vi "regresion_AB.vi"() -> ()   [LabVIEW 2025]
uses:
  <vilib>/Analysis/Matrix/Datatypes/RealMatrix.ctl
  <vilib>/Analysis/baseanly.llb/Mean (DBL).vi
  <vilib>/Analysis/baseanly.llb/Vector x A.vi
  <vilib>/Analysis/baseanly.llb/Real A x B.vi
  <vilib>/Utility/file.llb/Read Delimited Spreadsheet (DBL).vi
  <vilib>/Utility/file.llb/Read Delimited Spreadsheet (string).vi
  <vilib>/Analysis/Matrix/Numeric/Conversions/Array To Matrix - RA.vi
  <vilib>/Analysis/Matrix/Numeric/Add/Add - RM,RM.vi
  <vilib>/Analysis/Matrix/Numeric/Conversions/Matrix To Array - RM.vi
  <vilib>/Analysis/NI_AALBase.lvlib
  <vilib>/Analysis/Matrix/NI_Matrix.lvlib
  <vilib>/ptbypt/NI_PtbyPt.lvlib
panel:
  out "平滑化":dbl[](array[numeric])
  out "output array":dbl[][](array[numeric])
  out "圧力中心列_2":dbl[](graph)
  out "荷重N_2":dbl[](graph)
  out "平均圧力_2":dbl[](graph)
  out "圧力中心列_1":dbl[](graph)
  out "圧力中心行_1":dbl[](graph)
  out "荷重N_1(接触と似た形)":dbl[](graph)
  out "接触%_1":dbl[](graph)
  out "COPY Graph 3":dbl[](graph)
  out "COPX Graph":dbl[](graph)
  out "Real 2D Array":dbl[][](array[numeric])
  out "element 2":dbl
  out "element":dbl
  out "appended array":dbl[](array[numeric])
  out "python成形済み入力":dbl[](array[numeric])
  out "モデルA出力":T1
  out "モデルB入力":T1
  out "モデルB最終出力":T1
  out "Array 4":dbl[][](array[numeric])
  in  "stop":bool
  out "動画終了フラグ":bool
  out "input array":dbl[](array[numeric])
  out "op_magnitude":dbl
  out "steer_COPy":dbl
  out "steer_COPx":dbl
  out "pedal_COPy":dbl
  out "pedal_COPx":dbl
  out "COP_radius":dbl
  out "phys_torsion":dbl
  out "phys_roll":dbl
  out "phys_pitch":dbl
  out "COP_Y_phys":dbl
  out "+LR/2":dbl
  out "-LR/2":dbl
  out "-FR/2":dbl
  out "+FR/2":dbl
  out "COP_X_phys":dbl
  out "W":dbl
  out "ペダル（0index）":dbl[][](array[numeric])
  out "ペダルを踏んだ量 3":dynamicdata(graph)
  out "表示ループ9":i32
  out "緊急停止フラグ":bool
  out "モデルA重み":dbl[][](array[numeric])
  out "モデルAバイアス":dbl[][](array[numeric])
  out "モデルAオーダー":string[][](array[string])
  out "モデルA入力(最初)":dbl[][](array[numeric])
  out "モデルB重み":dbl[][](array[numeric])
  out "モデルBバイアス":dbl[][](array[numeric])
  # "17"
  # "17"
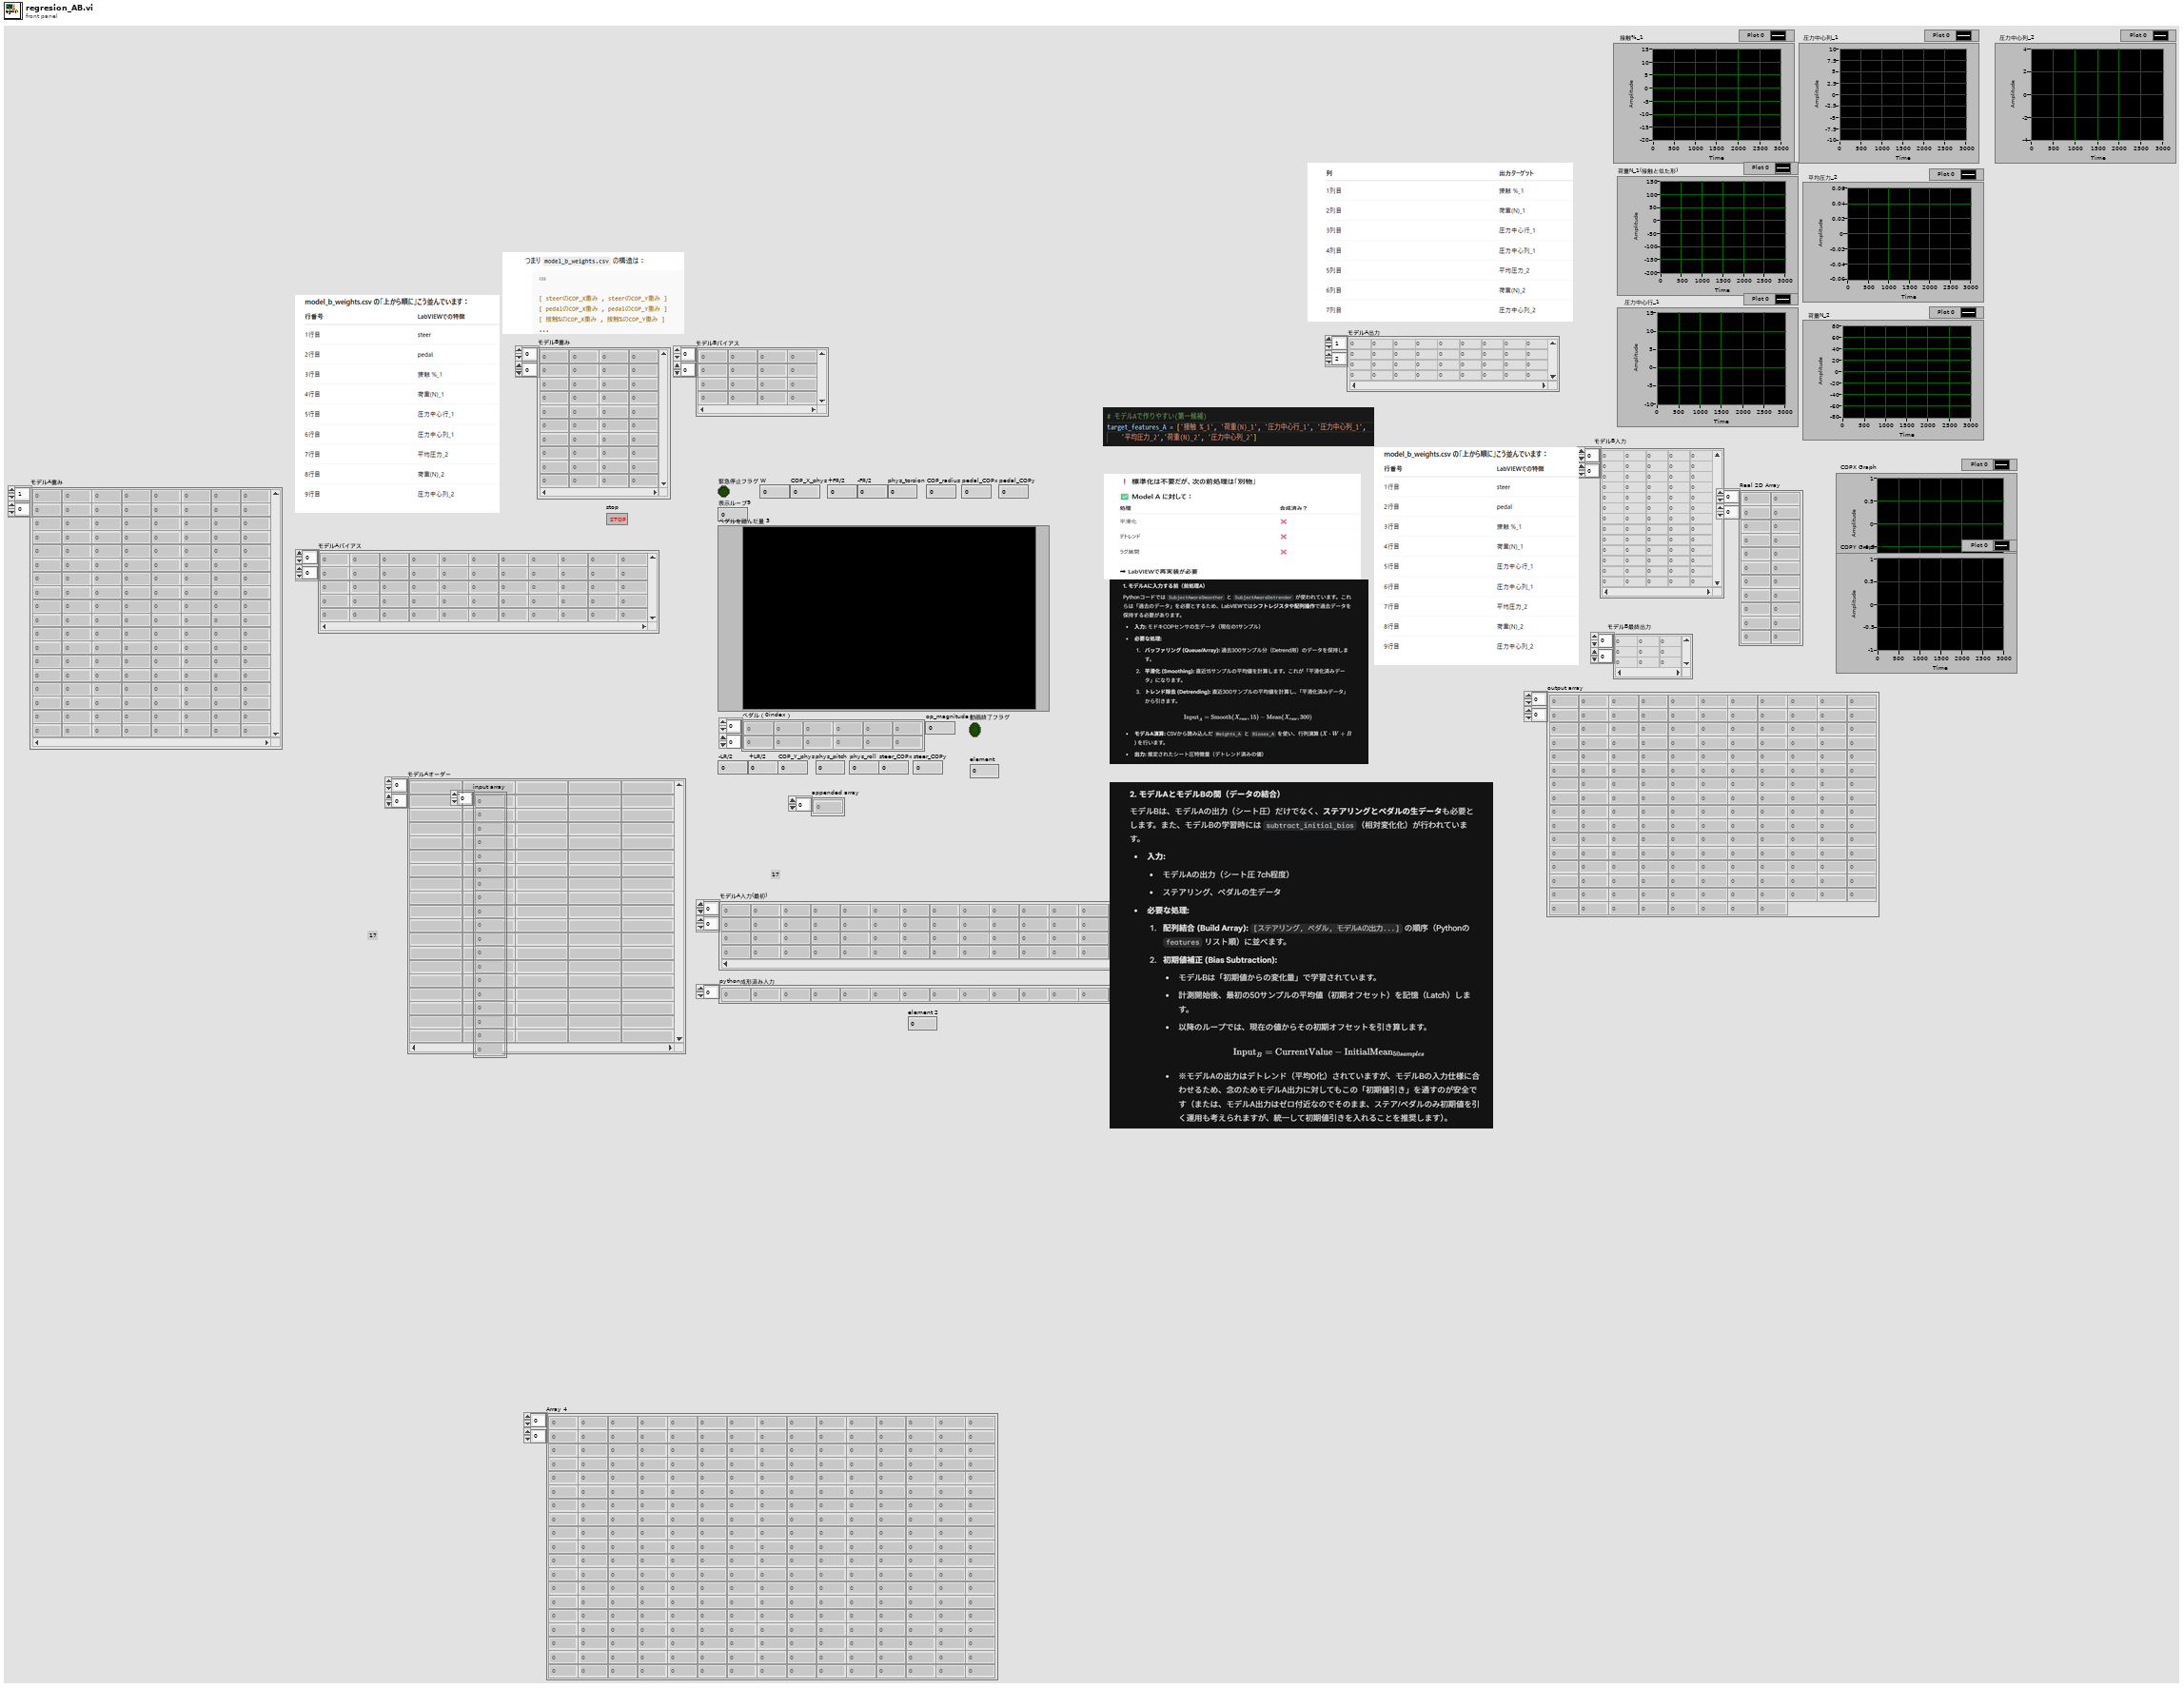
[diagram p1: front panel]
types:
  T1 = typedef "NI_Matrix.lvlib/RealMatrix.ctl" = dbl[][]
diagram:
  # "列 col"
  # "行 lag"
  # "モデルB"
  n1 = flat-sequence {
    tunnel: [w34] -> w25
    tunnel: [w33] -> w24
    tunnel: [w32] -> w23
    frame #0 {
      w39 = ","
      n2 = call <vilib>:"Application Directory.vi"() -> ("Application Directory"=w37:path)
      n3 = Build Path(base path=w37, name or relative path="学習済み") -> (appended path=w35:path)
      n4 = Build Path(base path=w35, name or relative path="model_a_biases.csv") -> (appended path=w44:path)
      n5 = Build Path(base path=w35, name or relative path="model_a_test_input.csv") -> (appended path=w43:path)
      n6 = Build Path(base path=w35, name or relative path="model_a_weights.csv") -> (appended path=w45:path)
      n7 = Build Path(base path=w35, name or relative path="model_a_test_output_expected.csv") -> (appended path=w42:path)
      n8 = Build Path(base path=w35, name or relative path="model_a_input_order.csv") -> (appended path=w40:path)
      n9 = call-poly <vilib>:"Read Delimited Spreadsheet.vi"("file path (dialog if empty)"=w45, "delimiter (\\t)"=w39) -> ("all rows"=w34:dbl[][])  [unwired: 8 in, 5 out]
      "モデルA重み" <- w34
      n10 = call-poly <vilib>:"Read Delimited Spreadsheet.vi"("file path (dialog if empty)"=w44, "delimiter (\\t)"=w39) -> ("all rows"=w33:dbl[][])  [unwired: 8 in, 5 out]
      "モデルAバイアス" <- w33
      n11 = call-poly <vilib>:"Read Delimited Spreadsheet.vi"("file path (dialog if empty)"=w43, "delimiter (\\t)"=w39) -> ("all rows"=w32:dbl[][])  [unwired: 8 in, 5 out]
      "モデルA入力(最初)" <- w32
      n12 = call-poly <vilib>:"Read Delimited Spreadsheet.vi"("file path (dialog if empty)"=w42, "delimiter (\\t)"=w39) -> ()  [unwired: 8 in, 6 out]
      n13 = call-poly <vilib>:"Read Delimited Spreadsheet.vi"("file path (dialog if empty)"=w40, "delimiter (\\t)"=w39) -> ("all rows"=→"モデルAオーダー":string[][])  [unwired: 8 in, 5 out]
    }
  }
  n14 = flat-sequence {
    tunnel: [w51] -> w27
    tunnel: [w50] -> w26
    frame #0 {
      w55 = ","
      n15 = call <vilib>:"Application Directory.vi"() -> ("Application Directory"=w54:path)
      n16 = Build Path(base path=w54, name or relative path="学習済み") -> (appended path=w52:path)
      n17 = Build Path(base path=w52, name or relative path="model_b_biases.csv") -> (appended path=w58:path)
      n18 = Build Path(base path=w52, name or relative path="model_b_test_output_expected.csv") -> (appended path=w56:path)
      n19 = Build Path(base path=w52, name or relative path="model_b_test_input.csv") -> (appended path=w57:path)
      n20 = Build Path(base path=w52, name or relative path="model_b_weights.csv") -> (appended path=w59:path)
      n21 = call-poly <vilib>:"Read Delimited Spreadsheet.vi"("file path (dialog if empty)"=w59, "delimiter (\\t)"=w55) -> ("all rows"=w51:dbl[][])  [unwired: 8 in, 5 out]
      "モデルB重み" <- w51
      n22 = call-poly <vilib>:"Read Delimited Spreadsheet.vi"("file path (dialog if empty)"=w58, "delimiter (\\t)"=w55) -> ("all rows"=w50:dbl[][])  [unwired: 8 in, 5 out]
      "モデルBバイアス" <- w50
      n23 = call-poly <vilib>:"Read Delimited Spreadsheet.vi"("file path (dialog if empty)"=w57, "delimiter (\\t)"=w55) -> ()  [unwired: 8 in, 6 out]
      n24 = call-poly <vilib>:"Read Delimited Spreadsheet.vi"("file path (dialog if empty)"=w56, "delimiter (\\t)"=w55) -> ()  [unwired: 8 in, 6 out]
    }
  }
  n25 = Initialize Array(0.0, 16, 14) -> (w28:dbl[][])
  n26 = for {
    shift-right: [w66] -> _
    shift-left: w28 -> [w92]
    tunnel: w27 -> [w82]
    tunnel: w26 -> [w83]
    tunnel: w25 -> [w90]
    tunnel: w24 -> [w89]
    tunnel: w23 -> [w78] mode=indexing
    tunnel: [w73] -> w21 mode=indexing
    tunnel: [w70] -> w12 mode=indexing
    i -> [w91]
    w99 = dbl[][] [[1.23, 3.5, 2.61, 3.01, 0.17, 0.19]] ("2DData")
    w100 = dbl[][] [[1.65, 3.5, 2.61, 3.01, 0.17, 0.19]] ("2DData")
    w152 = -1
    w154 = 2
    w116 = 0
    w97 = 0
    # "ステア"
    # "ペダル"
    # "30Hz"
    # "LR"
    # "FR"
    # "F4"
    # "F3"
    # "F2"
    # "F1"
    # "pedal_COPy"
    # "pedal_COPx"
    # "steer_COPy"
    # "steer_COPx"
    # "COP_angle"
    # "COP_radius"
    # "phys_torsion"
    # "phys_roll"
    # "phys_pitch"
    # "COP_Y_phys"
    # "COP_X_phys"
    # "W"
    n27 = Index Array(array=w78, index=7) -> (element=w76:dbl)
    "element" <- w76
    n28 = Index Array(array=w78, index=6) -> (element=w77:dbl)
    "element 2" <- w77
    n29 = Wait (ms)(milliseconds to wait=1.0) -> ()  [unwired: 1 out]
    n30 = call "Convert to Dynamic Data"("2D Array"=w99) -> ("Dynamic Data Type"=→"ペダルを踏んだ量 3":dynamicdata)  [unwired: 3 in]
    n31 = flat-sequence {
      tunnel: w90 -> [w168]
      tunnel: w89 -> [w166]
      tunnel: [w163] -> w86
      tunnel: w78 -> [w162]
      tunnel: w86 -> [w170]
      tunnel: w85 -> [_]
      tunnel: w84 -> [_]
      tunnel: [w173] -> w81
      tunnel: w77 -> [w172]
      tunnel: w76 -> [w171]
      tunnel: [w169] -> w71
      tunnel: w83 -> [w185]
      tunnel: w82 -> [w184]
      tunnel: w81 -> [w182]
      tunnel: [w179] -> w74
      frame #0 {
        n32 = call-poly <vilib>:"A x B.vi"("Matrix A"=w168, "Vector V'"=w162) -> ("V' x A"=w167:dbl[])  [unwired: 1 out]
        n33 = call-poly <vilib>:"Array To Matrix.vi"("Real 1D Array"=w167) -> ("Real Matrix (Column Vector)"=w165:T1)
        n34 = Transpose Matrix(1:w165) -> (0:w164:T1)
        n35 = call-poly <vilib>:"Add.vi"("Real Matrix B"=w166, "Real Matrix A"=w164) -> ("A + B"=w163:T1)
      }
      frame #1 {
        n36 = call-poly <vilib>:"Matrix To Array.vi"("Real Matrix"=w170) -> ("Real 2D Array"=w178:dbl[][])
        n37 = call-poly <vilib>:"Matrix To Array.vi"("Real Matrix"=w170) -> ("Real 2D Array"=w169:dbl[][])
        n38 = Index Array(array=w178, index (row)=0) -> (element=w176:dbl[])  [unwired: 1 in]
        n39 = Build Array (concatenate)(w172, w176) -> (w175:dbl[])
        n40 = Build Array (concatenate)(w171, w175) -> (w174:dbl[])
        n41 = call-poly <vilib>:"Array To Matrix.vi"("Real 1D Array"=w174) -> ("Real Matrix (Column Vector)"=w173:T1)
        "モデルB入力" <- w173
        "モデルA出力" <- w170
      }
      frame #2 {
        n42 = Transpose Matrix(1:w182) -> (0:w181:T1)
        n43 = call-poly <vilib>:"A x B.vi"("B"=w184, "A"=w181) -> ("A x B"=w183:T1)  [unwired: 1 out]
        n44 = call-poly <vilib>:"Add.vi"("Real Matrix B"=w185, "Real Matrix A"=w183) -> ("A + B"=w180:T1)
        "モデルB最終出力" <- w180
        n45 = call-poly <vilib>:"Matrix To Array.vi"("Real Matrix"=w180) -> ("Real 2D Array"=w179:dbl[][])
      }
    }
    n46 = Index Array(array=w100, index (row)=w116, index (col)=w116) -> (element=w115:dbl)
    n47 = Index Array(array=w100, index (row)=w116, index (col)=1) -> (element=w114:dbl)
    n48 = Index Array(array=w100, index (row)=w116, index (col)=2) -> (element=w113:dbl)
    n49 = Index Array(array=w100, index (row)=w116, index (col)=3) -> (element=w112:dbl)
    n50 = Index Array(array=w100, index (row)=w116, index (col)=4) -> ()  [unwired: 1 out]
    n51 = Index Array(array=w100, index (row)=w116, index (col)=5) -> ()  [unwired: 1 out]
    n52 = Index Array(array=dbl[][] [[90.0, 3.5, 2.61, 3.01, 0.17, 0.19]] ("2DData"), index (row)=w97, index (col)=w97) -> (element=w84:dbl)
    n53 = Index Array(array=w99, index (row)=w97, index (col)=w97) -> (element=w85:dbl)
    n54 = Divide(x=0.43, y=w154) -> (x/y=w141:dbl)
    "+LR/2" <- w141
    n55 = Divide(x=0.454, y=w154) -> (x/y=w149:dbl)
    "+FR/2" <- w149
    n56 = Multiply(x=w149, y=w152) -> (x*y=w148:dbl)
    "-FR/2" <- w148
    n57 = Multiply(x=w141, y=w152) -> (x*y=w140:dbl)
    "-LR/2" <- w140
    n58 = Add(x=w115, y=w114) -> (x+y=w158:dbl)
    n59 = Add(x=w158, y=w113) -> (x+y=w157:dbl)
    n60 = Add(x=w157, y=w112) -> (x+y=w134:dbl)
    "W" <- w134
    n61 = Delete From Array(array=w92, length=1, index (row)=15) -> (array with subset deleted=w95:dbl[][])  [unwired: 1 in, 1 out]
    n62 = Multiply(x=w115, y=w149) -> (x*y=w147:dbl)
    n63 = Multiply(x=w114, y=w149) -> (x*y=w146:dbl)
    n64 = Multiply(x=w115, y=w141) -> (x*y=w139:dbl)
    n65 = Multiply(x=w113, y=w148) -> (x*y=w145:dbl)
    n66 = Multiply(x=w114, y=w140) -> (x*y=w138:dbl)
    n67 = Multiply(x=w112, y=w148) -> (x*y=w144:dbl)
    n68 = Multiply(x=w113, y=w141) -> (x*y=w137:dbl)
    n69 = Multiply(x=w112, y=w140) -> (x*y=w136:dbl)
    n70 = Add(x=w147, y=w146) -> (x+y=w153:dbl)
    n71 = Add(x=w139, y=w138) -> (x+y=w143:dbl)
    n72 = Add(x=w153, y=w145) -> (x+y=w151:dbl)
    n73 = Index Array(array=w71, index (row)=0) -> (element=w70:dbl[])  [unwired: 1 in]
    n74 = Add(x=w143, y=w137) -> (x+y=w142:dbl)
    n75 = Add(x=w151, y=w144) -> (x+y=w150:dbl)
    n76 = Add(x=w142, y=w136) -> (x+y=w135:dbl)
    n77 = Divide(x=w150, y=w134) -> (x/y=w111:dbl)
    "COP_X_phys" <- w111
    n78 = Multiply(x=w111, y=w85) -> (x*y=w102:dbl)
    "pedal_COPx" <- w102
    n79 = Multiply(x=w111, y=w84) -> (x*y=w104:dbl)
    "steer_COPx" <- w104
    n80 = Divide(x=w135, y=w134) -> (x/y=w110:dbl)
    "COP_Y_phys" <- w110
    n81 = Multiply(x=w110, y=w85) -> (x*y=w101:dbl)
    "pedal_COPy" <- w101
    n82 = Multiply(x=w110, y=w84) -> (x*y=w103:dbl)
    "steer_COPy" <- w103
    n83 = Add(x=w115, y=w114) -> (x+y=w133:dbl)
    n84 = Add(x=w113, y=w112) -> (x+y=w132:dbl)
    n85 = Add(x=w115, y=w113) -> (x+y=w131:dbl)
    n86 = Subtract(x=w133, y=w132) -> (x-y=w108:dbl)
    "phys_pitch" <- w108
    n87 = Add(x=w114, y=w112) -> (x+y=w130:dbl)
    n88 = Add(x=w115, y=w112) -> (x+y=w129:dbl)
    n89 = Add(x=w114, y=w113) -> (x+y=w128:dbl)
    n90 = Subtract(x=w131, y=w130) -> (x-y=w107:dbl)
    "phys_roll" <- w107
    n91 = Subtract(x=w129, y=w128) -> (x-y=w106:dbl)
    "phys_torsion" <- w106
    n92 = Square(x=w85) -> (x^2=w124:dbl)
    n93 = Square(x=w84) -> (x^2=w123:dbl)
    n94 = Add(x=w124, y=w123) -> (x+y=w122:dbl)
    n95 = Square(x=w111) -> (x^2=w127:dbl)
    n96 = Square(x=w110) -> (x^2=w126:dbl)
    n97 = Square Root(x=w122) -> (sqrt(x)=w109:dbl)
    "op_magnitude" <- w109
    n98 = Add(x=w127, y=w126) -> (x+y=w125:dbl)
    n99 = Square Root(x=w125) -> (sqrt(x)=w105:dbl)
    "COP_radius" <- w105
    n100 = Build Array(w115, w114, w113, w112, w111, w110, w85, w84, w109, w108, w107, w106, w105, w104, w103, w102, w101) -> (w87:dbl[])
    "input array" <- w87
    "appended array" <- w87
    n101 = Insert Into Array(array=w95, index (row)=0, new element=w87) -> (w66:dbl[][])  [unwired: 1 in]
    "output array" <- w66
    n102 = Transpose 2D Array(2D array=w66) -> (transposed array=w65:dbl[][])
    n103 = for {
      tunnel: w65 -> [w161] mode=indexing
      tunnel: [w160] -> w64 mode=indexing
      n104 = call-poly <vilib>:"Mean.vi"("X"=w161) -> ("mean"=w160:dbl)  [unwired: 1 out]
    }
    "平滑化" <- w64
    n105 = call <vilib>:"Mean PtByPt.vi"("sample length"=15) -> ("mean"=w67:dbl)  [unwired: 3 in, 1 out]
    n106 = call <vilib>:"Mean PtByPt.vi"("x"=w67, "sample length"=3) -> ()  [unwired: 2 in, 2 out]
    n107 = Index Array(array=w74, index (row)=0) -> (element=w73:dbl[])  [unwired: 1 in]
    "表示ループ9" <- w91
    "ペダル（0index）" <- w99
    "Array 4" <- w92
    "python成形済み入力" <- w78
  }
  "Real 2D Array" <- w21
  n108 = Transpose 2D Array(2D array=w12) -> (transposed array=w1:dbl[][])
  n109 = Index Array(array=w1, index (row)=0) -> (element=→"接触%_1":dbl[])  [unwired: 1 in]
  n110 = Index Array(array=w1, index (row)=1) -> (element=→"荷重N_1(接触と似た形)":dbl[])  [unwired: 1 in]
  n111 = Index Array(array=w1, index (row)=4) -> (element=→"平均圧力_2":dbl[])  [unwired: 1 in]
  n112 = Index Array(array=w1, index (row)=3) -> (element=→"圧力中心列_1":dbl[])  [unwired: 1 in]
  n113 = Index Array(array=w1, index (row)=6) -> (element=→"圧力中心列_2":dbl[])  [unwired: 1 in]
  n114 = Index Array(array=w1, index (row)=2) -> (element=→"圧力中心行_1":dbl[])  [unwired: 1 in]
  n115 = Index Array(array=w1, index (row)=5) -> (element=→"荷重N_2":dbl[])  [unwired: 1 in]
  n116 = Transpose 2D Array(2D array=w21) -> (transposed array=w19:dbl[][])
  n117 = Index Array(array=w19, index (row)=0) -> (element=→"COPX Graph":dbl[])  [unwired: 1 in]
  n118 = Index Array(array=w19, index (row)=1) -> (element=→"COPY Graph 3":dbl[])  [unwired: 1 in]
